vi "testSharedVar.vi"   [LabVIEW 2013]
uses:
  <vilib>/CANopenLib/CANOPEN.llb/CANopen BaudRate.ctl
  <vilib>/CANopenLib/CANOPEN.llb/CANopen Interface Create.vi
  <vilib>/CANopenLib/CANOPEN.llb/CANopen SDO Create.vi
  <vilib>/CANopenLib/CANOPEN.llb/CANopen SDO Close.vi
  <vilib>/CANopenLib/CANOPEN.llb/CANopen Interface Close.vi
types:
  T1 = typedef "CANopen BaudRate.ctl" = u32
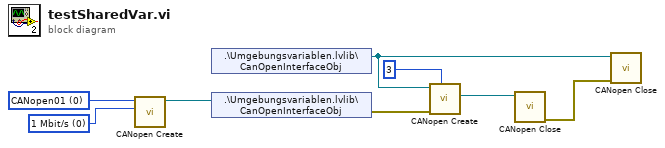
[diagram p0: block diagram]
diagram:
  w7 = T1 0 items=["1 Mbit/s"=0, "800 kbit/s"=1, "500 kbit/s"=2, "250 kbit/s"=3, "125 kbit/s"=4, "50 kbit/s"=6, "20 kbit/s"=7, "10 kbit/s"=8] ("baud rate")
  w8 = u32 0 items=["CANopen01", "CANopen02", "CANopen03", "CANopen04", "CANopen05", "CANopen06", "CANopen07", "CANopen08", "CANopen09", "CANopen10", "CANopen11", "CANopen12", "CANopen13", "CANopen14", "CANopen15", "CANopen16", "CANopen17", "CANopen18", "CANopen19", "CANopen20", "CANopen21", "CANopen22", "CANopen23", "CANopen24", "CANopen25", "CANopen26", "CANopen27", "CANopen28", "CANopen29", "CANopen30", "CANopen31", "CANopen32"] ("interface name")
  n1 = call-poly <vilib>:"CANopen Create.vi"("baud rate"=w7, "interface name"=w8) -> ("interface object out"=w6:refnum<k20>)  [unwired: 8 in, 1 out]
  n2 = shared-variable ".\\Umgebungsvariablen.lvlib\\CanOpenInterfaceObj"() -> (w1:refnum<k20>)  [unwired: 1 in, 1 out]
  n3 = shared-variable ".\\Umgebungsvariablen.lvlib\\CanOpenInterfaceObj"(w6) -> (error out=w5:errorcluster)  [unwired: 1 in]
  n4 = call-poly <vilib>:"CANopen Create.vi"("node-ID"=u8 3, "error in (no error)"=w5, "interface object in"=w1) -> ("SDO object out"=w3:refnum<k20>)  [unwired: 6 in, 2 out]
  n5 = call-poly <vilib>:"CANopen Close.vi"("SDO object in"=w3) -> ("error out"=w2:errorcluster)  [unwired: 10 in]
  n6 = call-poly <vilib>:"CANopen Close.vi"("error in (no error)"=w2, "interface object in"=w1) -> ()  [unwired: 9 in, 1 out]
